vi "Read Cycles and Mode.vi"(8 "error in (no error)":errorcluster, 11 "Auto UI in":refnum<class "Auto UI.lvclass">) -> (0 "error out":errorcluster, 2 "Cycles and Mode":refnum<vi>, 3 "Auto UI out":refnum<class "Auto UI.lvclass">)   [LabVIEW 2023, in "GUI.lvlib" / "Auto UI.lvlib" / "Auto UI.lvclass"]
uses:
  Auto UI.lvclass
  Typdefs/Auto GUI/Cycles and Mode.ctl
  Auto UI.lvclass/Auto UI.ctl
  GUI.lvlib
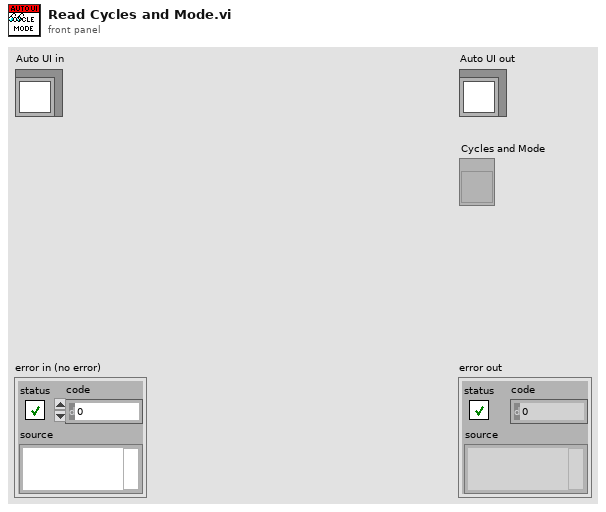
[diagram p1: front panel]
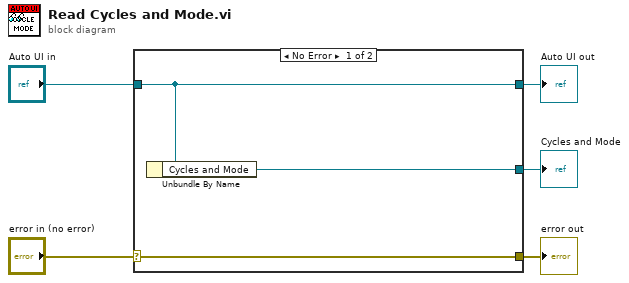
[diagram p0: block diagram]
diagram:
  n1 = case shown="No Error" "error in (no error)" {
    selector: "error in (no error)" -> [w8 w9]
    tunnel: [w8 w9] -> w4
    tunnel: [w7 w10] -> w2
    tunnel: "Auto UI in" -> [w7 w10]
    tunnel: [w6 _] -> w1
    frame No Error {
      n2 = Unbundle By Name(w7) -> ("Cycles and Mode"=w6:refnum<vi>)
    }
    frame Error {
    }
  }
  "error out" <- w4
  "Auto UI out" <- w2
  "Cycles and Mode" <- w1
